vi "ComputePath.vi"(9 "new goal reference":refnum<data-value>, 10 "current reference":refnum<data-value>, 11 "RVCLibrary_Bug2 in":refnum<class "RVCLibrary_Bug2.lvclass">) -> (3 "RVCLibrary_Bug2 out":refnum<class "RVCLibrary_Bug2.lvclass">)   [LabVIEW 2013, in "RVCLibrary_Bug2.lvclass"]
uses:
  RVCLibrary_Bug2.lvclass
  <vilib>/robotics/Navigation/shared/MapNode/AbstractDstarNode/NI_Robotics_AbstractDstarNode.lvclass
  <vilib>/robotics/Navigation/shared/WorldMap/AbstractWorldMap/NI_Robotics_AbstractWorldMap.lvclass
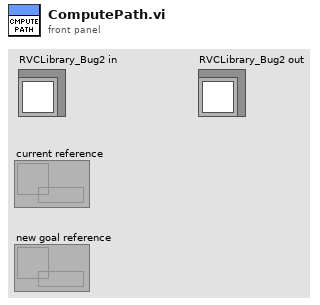
[diagram p1: front panel]
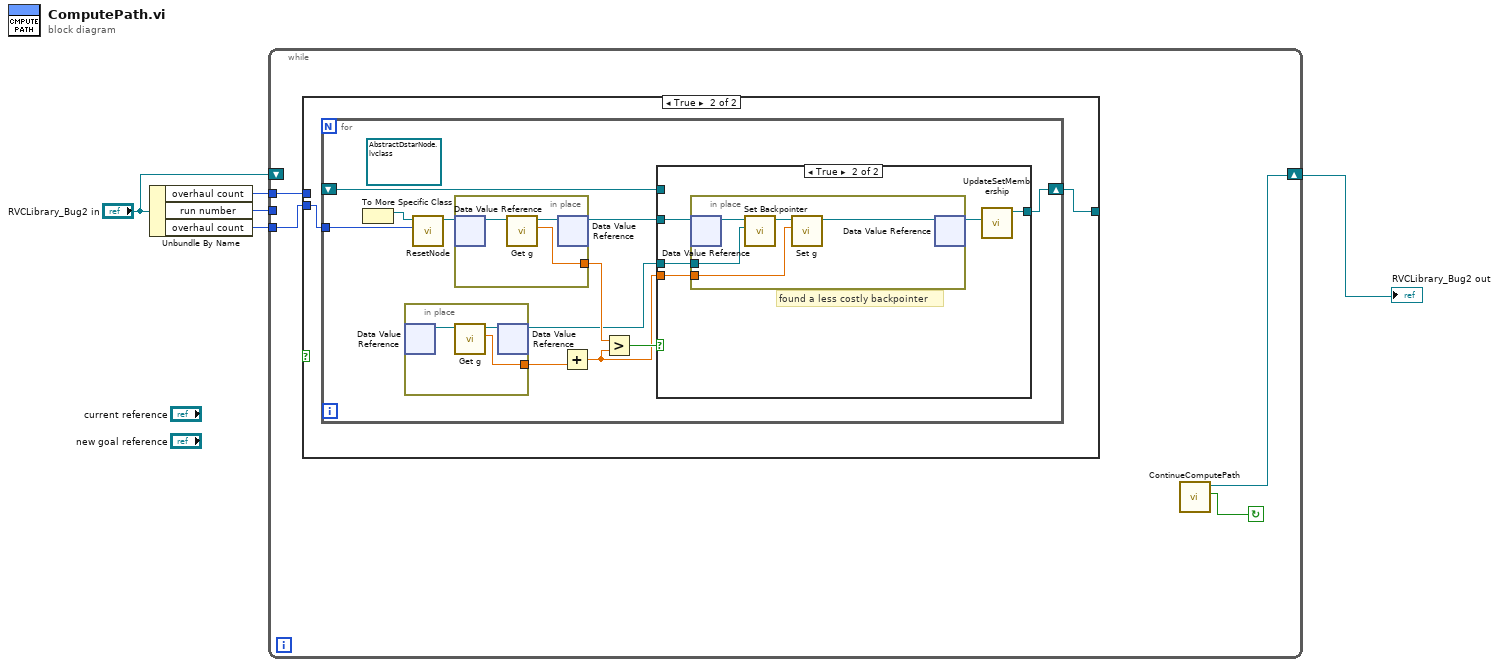
[diagram p0: block diagram]
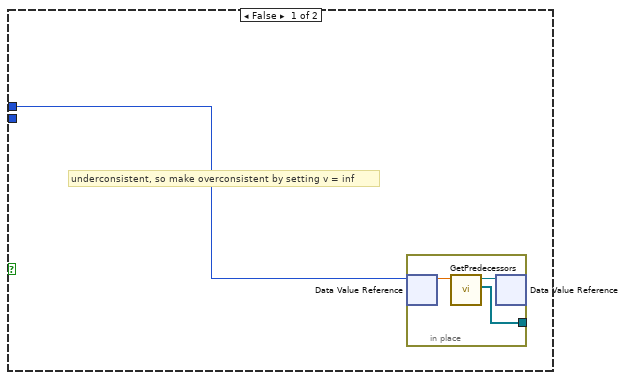
[diagram p2: hidden frame]
diagram:
  n1 = Unbundle By Name("RVCLibrary_Bug2 in") -> ("overhaul count"=w5:i32, "run number"=w3:i32, "overhaul count"=w4:i32)
  n2 = while {
    tunnel: w3 -> [_]
    tunnel: w5 -> [w9]
    shift-right: [w6] -> w2
    shift-left: "RVCLibrary_Bug2 in" -> [_]
    tunnel: w4 -> [w8]
    stop <- w7 continue-if-true
    n3 = case shown="True" {
      selector: _ -> [_ _]
      tunnel: [_ w15] -> _
      tunnel: w9 -> [w10 _]
      tunnel: w8 -> [_ w14]
      frame False {
        # "underconsistent, so make overconsistent by setting v = inf"
        n4 = in-place {
          in-place-border: [w11] -> _
          n5 = in-place-dvr #1(w10) -> (w13:dbl)  [unwired: 1 out]
          n6 = call-dynamic "GetPredecessors.vi"("WorldMap in"=w13) -> ("Predecessors"=w11:refnum<data-value>[], "WorldMap out"=w12:refnum<class "NI_Robotics_AbstractWorldMap.lvclass">)  [unwired: 7 in, 2 out]
          n7 = in-place-dvr #1(w12) -> ()  [unwired: 2 out]
        }
      }
      frame True {
        n8 = for {
          shift-right: [w20] -> w15
          shift-left: _ -> [w21]
          tunnel: w14 -> [w18]
          (unwired) refnum<data-value> refnum ("data value reference")
          n9 = To More Specific Class() -> (specific class reference=w17:refnum<data-value>)  [unwired: 3 in, 1 out]
          n10 = in-place {
            in-place-border: [w38] -> w19
            n11 = in-place-dvr #2() -> (w40:refnum<class "NI_Robotics_AbstractDstarNode.lvclass">)  [unwired: 1 in, 1 out]
            n12 = call <vilib>:"Get g.vi"("AbstractDstarNode in"=w40) -> ("g"=w38:dbl, "AbstractDstarNode out"=w39:refnum<class "NI_Robotics_AbstractDstarNode.lvclass">)  [unwired: 9 in]
            n13 = in-place-dvr #2(w39) -> (w23:refnum<data-value>)  [unwired: 1 out]
          }
          n14 = call "ResetNode.vi"("overhaul count"=w18, "node reference in"=w17) -> ("node reference out"=w16:refnum<data-value>)  [unwired: 9 in]
          n15 = in-place {
            in-place-border: [w41] -> w26
            n16 = in-place-dvr #3(w16) -> (w43:refnum<class "NI_Robotics_AbstractDstarNode.lvclass">)  [unwired: 1 out]
            n17 = call <vilib>:"Get g.vi"("AbstractDstarNode in"=w43) -> ("g"=w41:dbl, "AbstractDstarNode out"=w42:refnum<class "NI_Robotics_AbstractDstarNode.lvclass">)  [unwired: 9 in]
            n18 = in-place-dvr #3(w42) -> (w24:refnum<data-value>)  [unwired: 1 out]
          }
          n19 = Add(y=w19) -> (x+y=w22:dbl)  [unwired: 1 in]
          n20 = Greater?(x=w26, y=w22) -> (0:w25:bool)
          n21 = case shown="True" w25 {
            tunnel: w24 -> [_ w32]
            tunnel: w23 -> [_ w28]
            tunnel: w22 -> [_ w31]
            tunnel: w21 -> [w27 _]
            tunnel: [w27 w29] -> w20
            frame False {
              # "neighbor's current bp is less costly, so leave alone"
            }
            frame True {
              # "found a less costly backpointer"
              n22 = in-place {
                in-place-border: w28 -> [w36]
                in-place-border: w31 -> [w35]
                n23 = in-place-dvr #4(w32) -> (w37:refnum<class "NI_Robotics_AbstractDstarNode.lvclass">)  [unwired: 1 out]
                n24 = call <vilib>:"Set Backpointer.vi"("BackPointer"=w36, "AbstractDstarNode in"=w37) -> ("AbstractDstarNode out"=w34:refnum<class "NI_Robotics_AbstractDstarNode.lvclass">)  [unwired: 8 in, 1 out]
                n25 = call <vilib>:"Set g.vi"("g"=w35, "AbstractDstarNode in"=w34) -> ("AbstractDstarNode out"=w33:refnum<class "NI_Robotics_AbstractDstarNode.lvclass">)  [unwired: 9 in]
                n26 = in-place-dvr #4(w33) -> (w30:refnum<data-value>)  [unwired: 1 out]
              }
              n27 = call "UpdateSetMembership.vi"("node ref in"=w30) -> ("RVCLibrary_Bug out"=w29:refnum<class "RVCLibrary_Bug2.lvclass">)  [unwired: 9 in, 1 out]
            }
          }
        }
      }
    }
    n28 = call "ContinueComputePath.vi"() -> ("continue computing path"=w7:bool, "RVCLibrary_Bug2 out"=w6:refnum<class "RVCLibrary_Bug2.lvclass">)  [unwired: 10 in]
  }
  "RVCLibrary_Bug2 out" <- w2
